vi "Reparent Element.vi"(7 "New Parent":refnum<class "Config Element.lvclass">, 8 "error in (no error)":errorcluster, 10 "Element":refnum<class "Config Element.lvclass">, 11 "Config Manager in":refnum<class "Config Manager.lvclass">) -> (0 "error out":errorcluster, 3 "Config Manager out":refnum<class "Config Manager.lvclass">)   [LabVIEW 2023, in "CDM-Config.lvlib" / "Config Manager.lvclass"]
uses:
  Config Manager.lvclass
  Config Element/Config Element.lvclass
  Config Manager.lvclass/Config Manager.ctl
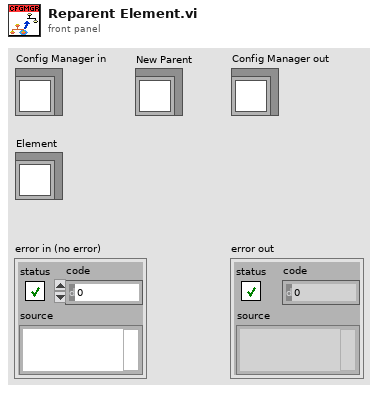
[diagram p1: front panel]
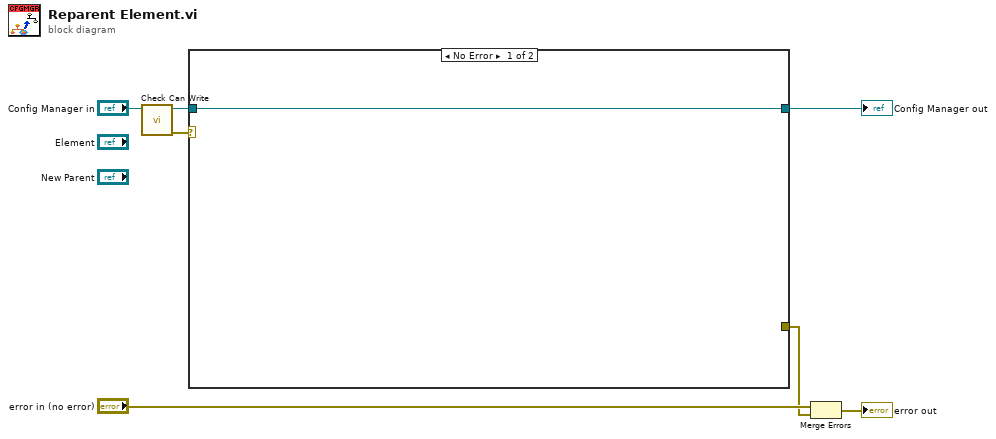
[diagram p0: block diagram]
diagram:
  n1 = call "Check Can Write.vi"("Config Manager in"="Config Manager in") -> ("error out"=w4:errorcluster, "Config Manager out"=w5:refnum<class "Config Manager.lvclass">)  [unwired: 9 in]
  n2 = case shown="No Error" w4 {
    selector: w4 -> [_ w9]
    tunnel: [w8 w10] -> w6
    tunnel: w5 -> [w8 w10]
    tunnel: [_ w9] -> w1
    frame No Error {
    }
    frame Error {
    }
  }
  "Config Manager out" <- w6
  n3 = Merge Errors("error in (no error)", w1) -> (→"error out":errorcluster)
